vi "GetBufferAppendMode.vi"(7 "SMU":T1, 8 "Error In":errorcluster, 10 "Buffer":u8=1 min=1 max=2 step=1, 11 "Kiethley 2602 In":refnum<visa-resource-name>) -> (0 "Error Out":errorcluster, 2 "Enabled?":bool, 3 "Keithley 2602 Out":refnum<visa-resource-name>)   [LabVIEW 2012, in "Keithley-2602.lvlib"]
uses:
  Keithley-2602.lvlib
  Controls/SMU.ctl
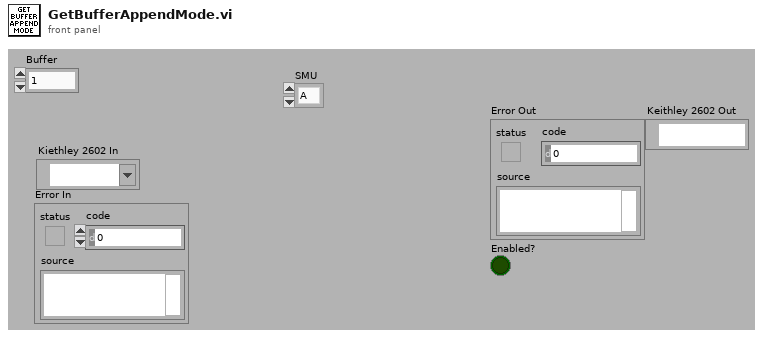
[diagram p1: front panel]
types:
  T1 = typedef "Keithley-2602.lvlib/SMU.ctl" = enum16{"A", "B"}
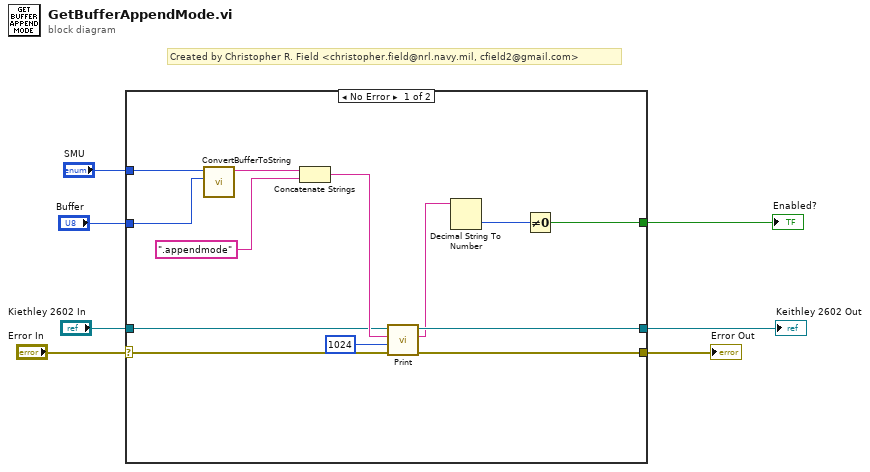
[diagram p0: block diagram]
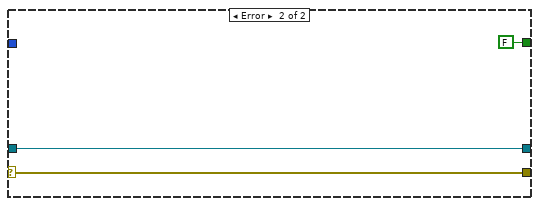
[diagram p2: hidden frame]
diagram:
  # "Created by Christopher R. Field <christopher.field@nrl.navy.mil, cfield2@gmail.com>"
  n1 = case shown="No Error" "Error In" {
    selector: "Error In" -> [w8 w22]
    tunnel: "Kiethley 2602 In" -> [w18 w23]
    tunnel: [w17 w22] -> w6
    tunnel: [w16 w23] -> w5
    tunnel: [w13 FALSE] -> w4
    tunnel: "Buffer" -> [w12 _]
    tunnel: "SMU" -> [w9 _]
    frame No Error {
      n2 = call "ConvertBufferToString.vi"("Buffer"=w12, "SMU"=w9) -> ("Buffer"=w11:string)  [unwired: 9 in]
      n3 = Concatenate Strings(w11, ".appendmode" ("string")) -> (w20:string)
      n4 = call "Print.vi"("Error In"=w8, "Byte Count"=u32 1024, "Attribute"=w20, "Kiethley 2602 In"=w18) -> ("Error Out"=w17:errorcluster, "Output"=w15:string, "Keithley 2602 Out"=w16:refnum<visa-resource-name>)  [unwired: 5 in]
      n5 = Decimal String To Number(string=w15) -> (number=w14:i32)  [unwired: 2 in, 1 out]
      n6 = Not Equal To 0?(x=w14) -> (x != 0?=w13:bool)
    }
    frame Error {
    }
  }
  "Error Out" <- w6
  "Keithley 2602 Out" <- w5
  "Enabled?" <- w4
